vi "close1D.vi"(8 "error in (no error)":errorcluster, 11 "xml":refnum<class "NativeXML.lvclass">[](array[class])) -> (0 "error out":errorcluster)   [LabVIEW 2009]
uses:
  NativeXML.lvclass
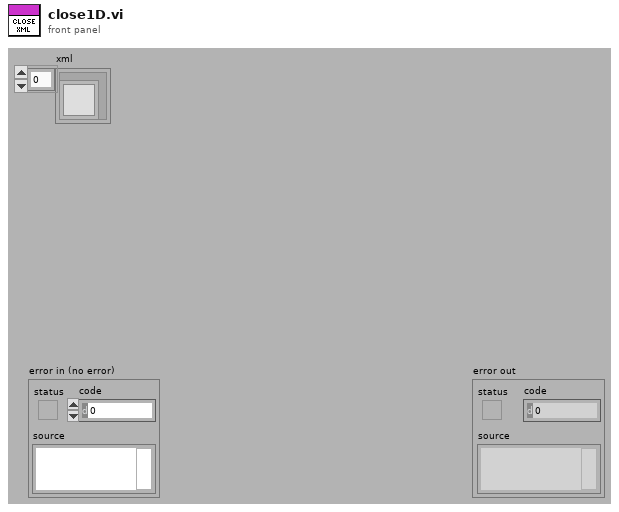
[diagram p1: front panel]
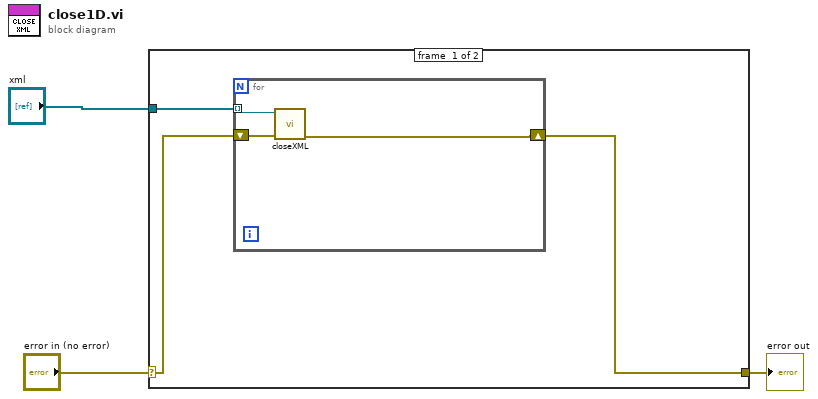
[diagram p0: block diagram]
diagram:
  n1 = case shown="No Error" "error in (no error)" {
    selector: "error in (no error)" -> [w5 w10]
    tunnel: [w4 w10] -> w2
    tunnel: "xml" -> [w6 _]
    frame #0 {
      n2 = for {
        tunnel: w6 -> [w8] mode=indexing
        shift-right: [w7] -> w4
        shift-left: w5 -> [w9]
        n3 = call "closeXML.vi"("error in (no error)"=w9, "NativeXML in"=w8) -> ("error out"=w7:errorcluster)  [unwired: 9 in]
      }
    }
    frame #1 {
    }
  }
  "error out" <- w2
